vi "convert_joinFieldData.vi"(0 "Parameters":string[](array[string]), 3 "Variables":string[](array[string])) -> (14 "Result List":string[](array[string]), 17 "Result String":string)   [LabVIEW 2018, in "db_lib R3.lvlib"]
uses:
  db_lib R3.lvlib
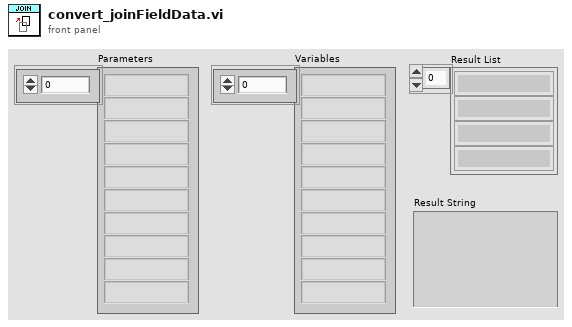
[diagram p1: front panel]
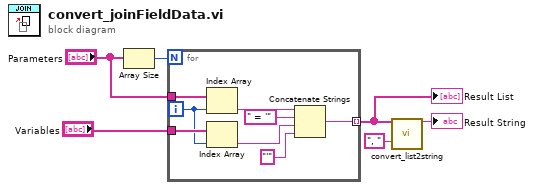
[diagram p0: block diagram]
diagram:
  n1 = Array Size(array="Parameters") -> (size(s)=w6:i32)
  n2 = for {
    N: w6 -> [_]
    tunnel: "Parameters" -> [w14]
    tunnel: "Variables" -> [w13]
    tunnel: [w7] -> w3 mode=indexing
    i -> [w12]
    n3 = Index Array(array=w14, index=w12) -> (element=w11:string)
    n4 = Index Array(array=w13, index=w12) -> (element=w9:string)
    n5 = Concatenate Strings(w11, " = '", w9, "'") -> (w7:string)
  }
  "Result List" <- w3
  n6 = call "convert_list2string.vi"("LIST"=w3, "SEPARATOR (CHAR)"=", " ("Separator")) -> ("RESULT"=→"Result String":string)  [unwired: 17 in]
